vi "Update DDS Arb Buffer.vi"(9 "arb_buffer_length":u32, 10 "arb_buffer":u16, 11 "channel_index":u8) -> (2 "arb_buffer out":u16)   [LabVIEW 2021, in "vmmso.lvlib"]
doc: "DLL_API void WINAPI UpdateDDSArbBuffer(unsigned char channel_index, unsigned short* arb_buffer, unsigned int arb_buffer_length);"
uses:
  vmmso.lvlib
  vmmso.dll
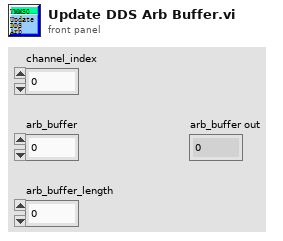
[diagram p1: front panel]
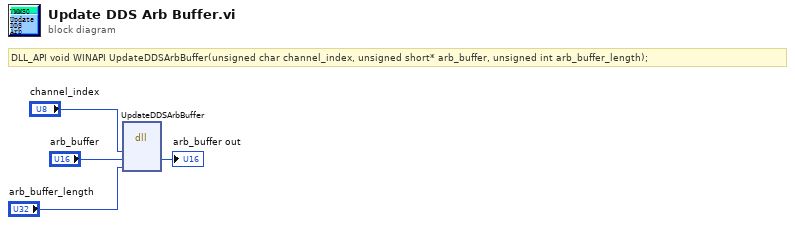
[diagram p0: block diagram]
diagram:
  # "DLL_API void WINAPI UpdateDDSArbBuffer(unsigned char channel_index, unsigned short* arb_buffer, unsigned int arb_buffer_length);"
  n1 = dll-call lib="D:/labviewdemo/LabviewDemo 21/vmmso/vmmso.*" fn="UpdateDDSArbBuffer"("channel_index"="channel_index", "arb_buffer"="arb_buffer", "arb_buffer_length"="arb_buffer_length") -> ("arb_buffer"=→"arb_buffer out":u16)  [unwired: 6 in, 2 out]
